vi "MouseOverEvent.vi"(0 "reference in":refnum<class "SparkLine.lvclass">, 5 "error in (no error)":errorcluster) -> (14 "reference out":refnum<class "SparkLine.lvclass">, 19 "error out":errorcluster)   [LabVIEW 2019, in "SparkLine.lvclass"]
uses:
  SparkLine.lvclass
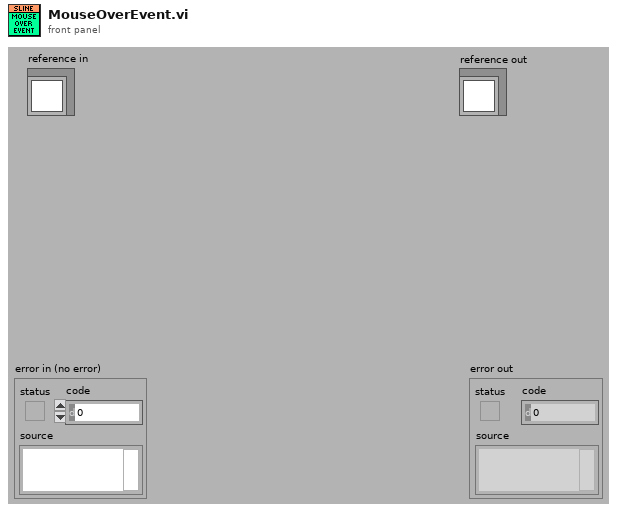
[diagram p1: front panel]
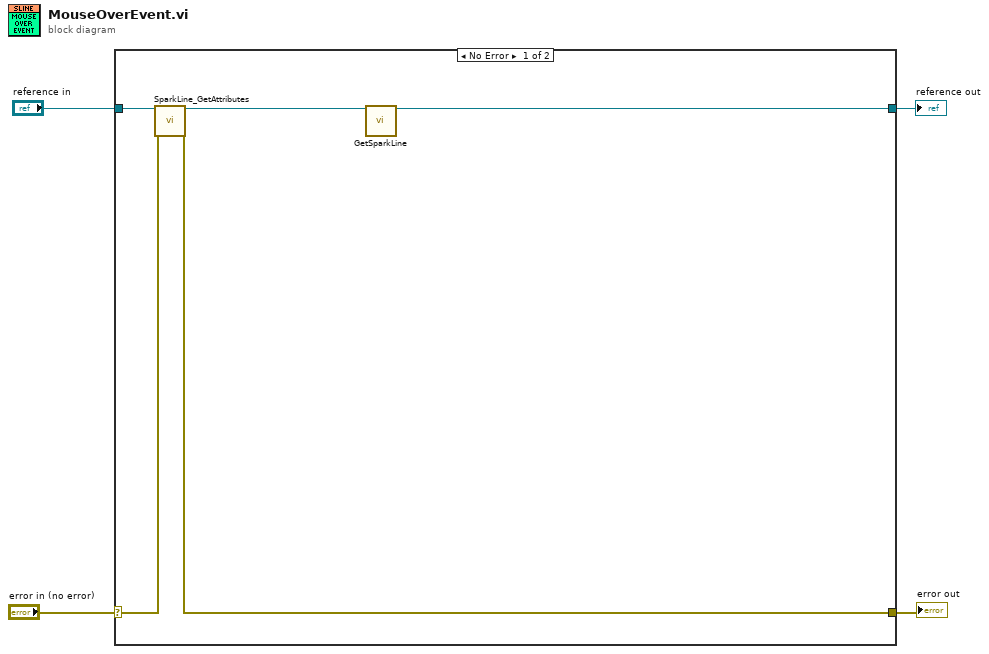
[diagram p0: block diagram]
diagram:
  n1 = case shown="No Error" "error in (no error)" {
    selector: "error in (no error)" -> [w9 w11]
    tunnel: [w8 w11] -> w3
    tunnel: [w5 w10] -> w1
    tunnel: "reference in" -> [w7 w10]
    frame No Error {
      n2 = call "SparkLine_GetAttributes.vi"("reference in"=w7, "error in (no error)"=w9) -> ("reference out"=w6:refnum<class "SparkLine.lvclass">, "error out"=w8:errorcluster)  [unwired: 14 in, 2 out]
      n3 = call-dynamic "GetSparkLine.vi"("reference in"=w6) -> ("reference out"=w5:refnum<class "SparkLine.lvclass">)  [unwired: 17 in, 1 out]
    }
    frame Error {
    }
  }
  "error out" <- w3
  "reference out" <- w1
